vi "[subVI]_time_delay.vi"(8 "milliseconds to wait":u32, 11 "error in":errorcluster) -> (3 "error out":errorcluster)   [LabVIEW 2013]
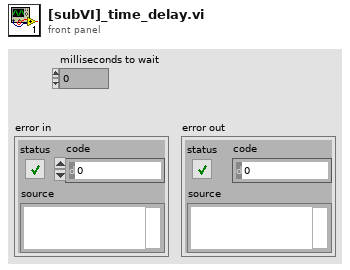
[diagram p1: front panel]
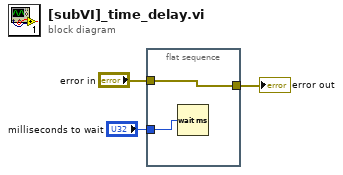
[diagram p0: block diagram]
diagram:
  n1 = flat-sequence {
    tunnel: "milliseconds to wait" -> [w5]
    tunnel: [w4] -> w2
    tunnel: "error in" -> [w4]
    frame #0 {
      n2 = Wait (ms)(milliseconds to wait=w5) -> ()  [unwired: 1 out]
    }
  }
  "error out" <- w2
